vi "Init Msg.vi"(6 "Teller":refnum<class "Teller.lvclass">, 9 "Parent Stopped":bool, 10 "Safe Stop":bool=TRUE) -> (3 "Stop Msg out":refnum<class "--Stop Msg.lvclass">)   [LabVIEW 2025, in "jettl.lvlib" / "Stop jettl Msg.lvlib" / "--Stop Msg.lvclass"]
uses:
  --Stop Msg.lvclass
  Teller/Teller.lvclass
  --Stop Msg.lvclass/--Stop Msg.ctl
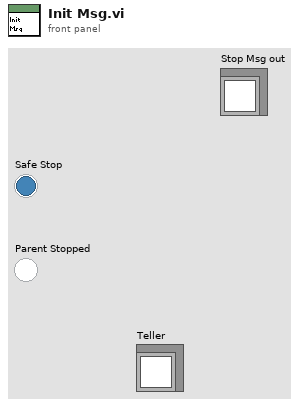
[diagram p1: front panel]
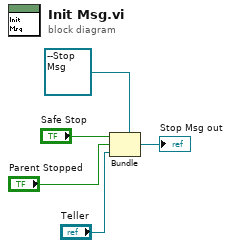
[diagram p0: block diagram]
diagram:
  n1 = Bundle "Bundle"(cluster=refnum<class "--Stop Msg.lvclass"> refnum ("Destroy Msg in"), "Safe Stop", "Parent Stopped", "Teller") -> (→"Stop Msg out":refnum<class "--Stop Msg.lvclass">)
